vi "OnDataChange.vi"(0 "GRMActor in":refnum<class "FlatField.lvclass">, 1 "DataExchange":T1, 3 "error in (no error)":errorcluster) -> (7 "GRMActor out":refnum<class "FlatField.lvclass">, 10 "error out":errorcluster)   [LabVIEW 2020, in "FlatField.lvlib" / "FlatField.lvclass"]
uses:
  FlatField.lvclass
  Hardware Abstraction Layer/Component/Device/Device/DataExchange.ctl
  Displayer/Displayer/FlatField Method.ctl
  FlatField.lvclass/FlatField.ctl
  Interface/DataListener Messages/OnDataChange Msg/OnDataChange Msg.lvclass/OnDataChange Msg.ctl
  <vilib>/ActorFramework/Message Enqueuer/Message Enqueuer.lvclass/Message Enqueuer.ctl
  FlatField Status.ctl
  <vilib>/ActorFramework/Message Enqueuer/Enqueue.vi
  Interface/DataListener Messages/OnDataChange Msg/OnDataChange Msg.lvclass
  C:/Program Files/National Instruments/LabVIEW 2020/vi.lib/ActorFramework/Message/Message.lvclass
  <vilib>/ActorFramework/Message Priority Queue/Priority Enqueue.vi
  Hardware Abstraction Layer/Component/GenericActor/GenericActor/GenericActor.lvclass
  Interface/DataListener/DataListener.lvclass
  <vilib>/vision/NI_Vision_Development_Module.lvlib
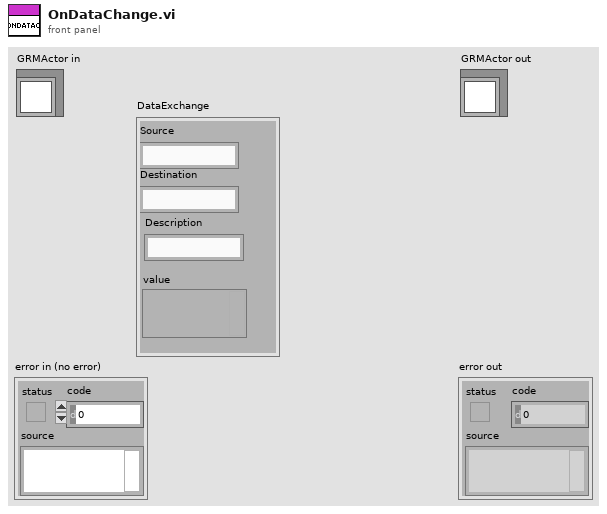
[diagram p1: front panel]
types:
  T1 = typedef "DataListener.lvclass/DataExchange.ctl" = cluster{"Source":string, "Destination":string, "Description":string, "value":variant}
  T2 = typedef "FlatField.lvlib/FlatField.lvclass/FlatField Method.ctl" = i32
  T3 = typedef "IMAQ Image.ctl" = refnum<image>
  T4 = typedef "FlatField.lvlib/FlatField.lvclass/FlatField Status.ctl" = i32
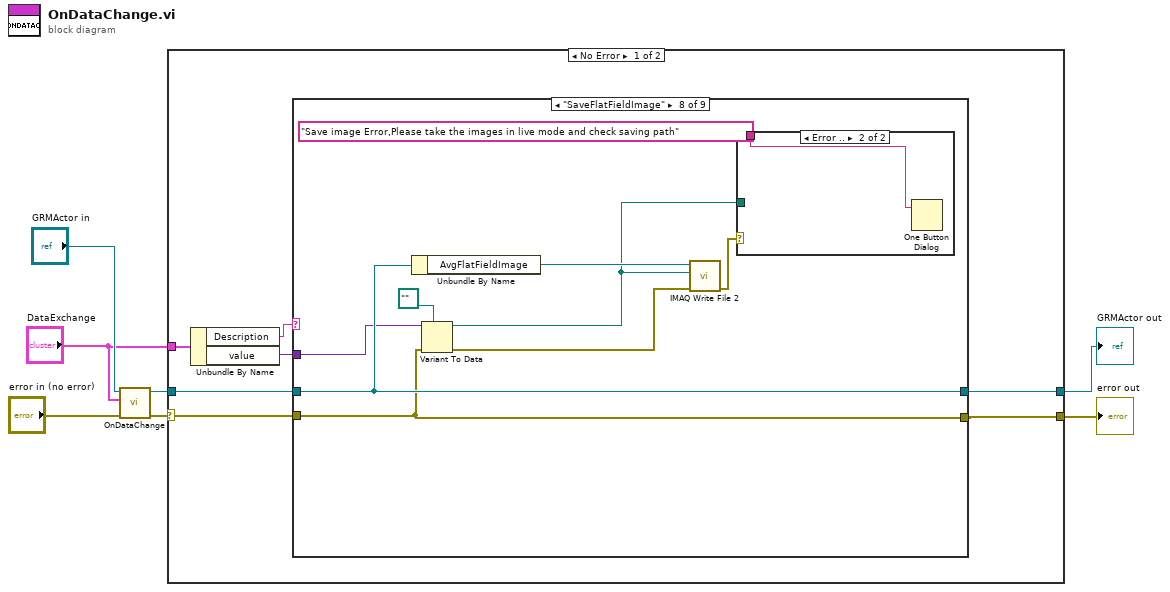
[diagram p0: block diagram]
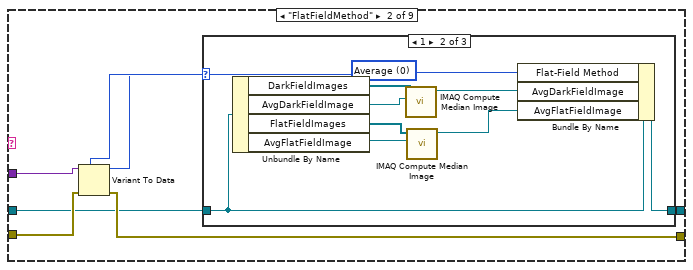
[diagram p3: hidden frame]
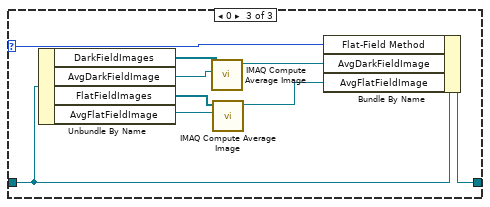
[diagram p5: hidden frame]
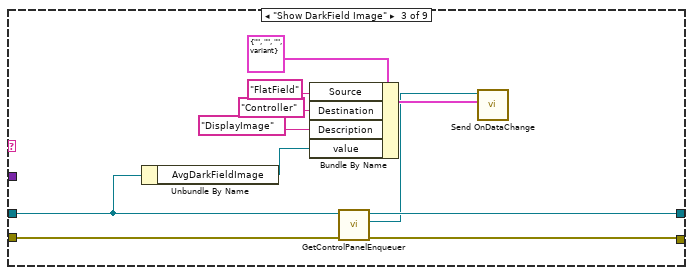
[diagram p6: hidden frame]
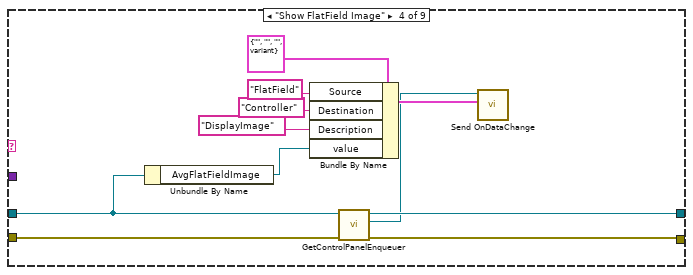
[diagram p7: hidden frame]
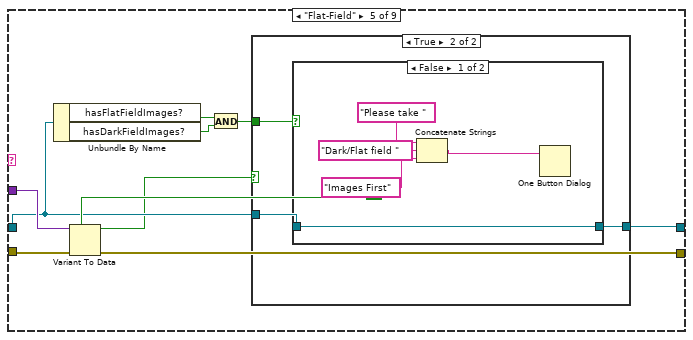
[diagram p8: hidden frame]
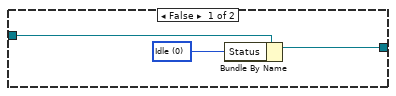
[diagram p9: hidden frame]
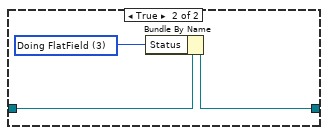
[diagram p10: hidden frame]
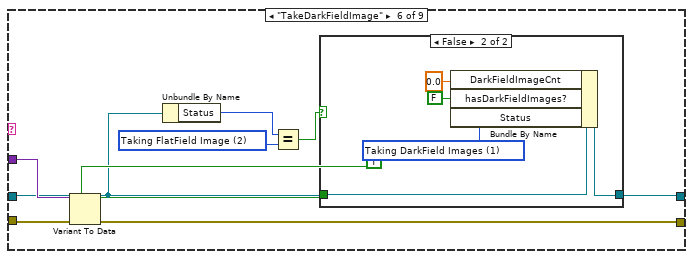
[diagram p11: hidden frame]
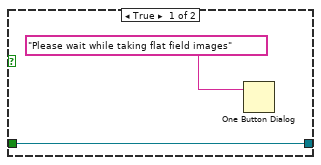
[diagram p12: hidden frame]
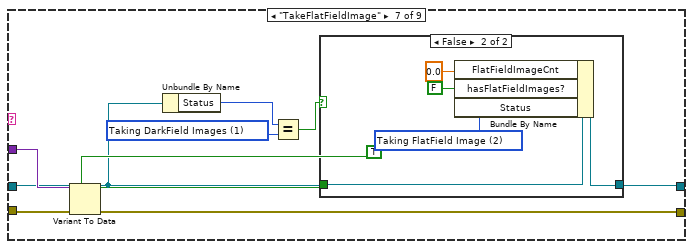
[diagram p13: hidden frame]
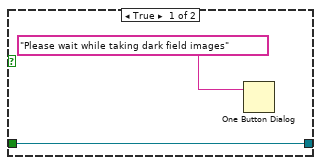
[diagram p14: hidden frame]
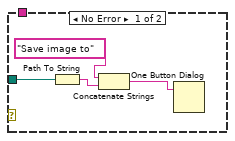
[diagram p15: hidden frame]
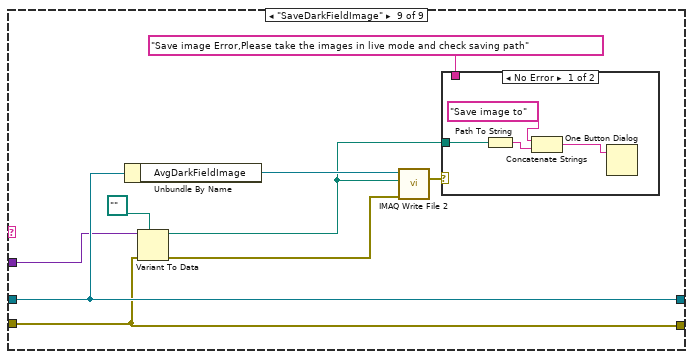
[diagram p16: hidden frame]
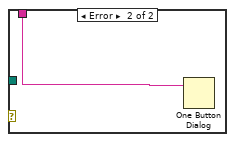
[diagram p17: hidden frame]
diagram:
  n1 = call-parent "OnDataChange.vi"("GRMActor in"="GRMActor in", "DataExchange"="DataExchange", "error in (no error)"="error in (no error)") -> ("GRMActor out"=w3:refnum<class "FlatField.lvclass">, "error out"=w5:errorcluster)  [unwired: 6 in]
  n2 = case shown="No Error" w5 {
    selector: w5 -> [w10 w151]
    tunnel: [w9 w151] -> w4
    tunnel: [w8 w152] -> w2
    tunnel: w3 -> [w11 w152]
    tunnel: "DataExchange" -> [w14 _]
    frame No Error {
      n3 = Unbundle By Name(w14) -> ("Description"=w13:string, "value"=w12:variant)
      n4 = case shown="\"SaveFlatFieldImage\"" w13 {
        tunnel: w12 -> [_ w20 _ _ w72 w96 w113 w129 w143]
        tunnel: [w16 w19 w46 w57 w70 w94 w111 w131 w145] -> w8
        tunnel: w11 -> [w16 w18 w44 w55 w69 w92 w109 w131 w145]
        tunnel: [w15 w22 w47 w58 w73 w97 w114 w125 w139] -> w9
        tunnel: w10 -> [w15 w23 w53 w64 w74 w98 w115 w125 w139]
        frame Default {
        }
        frame "FlatFieldMethod" {
          w21 = T2 0 items=["Average", "Median"] ("Flat-Field Method")
          n5 = Variant To Data(error in=w23, type=w21, Variant=w20) -> (data=w17:T2, error out=w22:errorcluster)
          n6 = case shown="1" w17 {
            selector: w17 -> [_ w31 w40]
            tunnel: [w24 w33 w42] -> w19
            tunnel: w18 -> [w24 w32 w41]
            frame Default {
            }
            frame 1 {
              n7 = Unbundle By Name(w32) -> ("DarkFieldImages"=w30:T3[], "AvgDarkFieldImage"=w29:T3, "FlatFieldImages"=w27:T3[], "AvgFlatFieldImage"=w26:T3)
              n8 = call "IMAQ Compute Median Image"("Image Dst"=w29, "Images"=w30) -> ("Image Dst Out"=w28:T3)  [unwired: 8 in, 1 out]
              n9 = call "IMAQ Compute Median Image"("Image Dst"=w26, "Images"=w27) -> ("Image Dst Out"=w25:T3)  [unwired: 8 in, 1 out]
              n10 = Bundle By Name(cluster=w32, "Flat-Field Method"=w31, "AvgDarkFieldImage"=w28, "AvgFlatFieldImage"=w25) -> (w33:refnum<class "FlatField.lvclass">)
            }
            frame 0 {
              n11 = Unbundle By Name(w41) -> ("DarkFieldImages"=w39:T3[], "AvgDarkFieldImage"=w38:T3, "FlatFieldImages"=w36:T3[], "AvgFlatFieldImage"=w35:T3)
              n12 = call "IMAQ Compute Average Image"("Image Dst"=w38, "Images"=w39) -> ("Image Dst Out"=w37:T3)  [unwired: 8 in, 1 out]
              n13 = call "IMAQ Compute Average Image"("Image Dst"=w35, "Images"=w36) -> ("Image Dst Out"=w34:T3)  [unwired: 8 in, 1 out]
              n14 = Bundle By Name(cluster=w41, "Flat-Field Method"=w40, "AvgDarkFieldImage"=w37, "AvgFlatFieldImage"=w34) -> (w42:refnum<class "FlatField.lvclass">)
            }
          }
        }
        frame "Show DarkField Image" {
          n15 = Unbundle By Name(w44) -> ("AvgDarkFieldImage"=w43:T3)
          n16 = Bundle By Name(cluster=T1 {"Source"="", "Destination"="", "Description"="", "value"=variant} ("DataExchange"), "Source"="FlatField", "Destination"="Controller", "Description"="DisplayImage", "value"=w43) -> (w51:T1)
          n17 = call-dynamic "GetControlPanelEnqueuer.vi"("error in (no error)"=w53, "GRMActor in"=w44) -> ("error out"=w47:errorcluster, "ControlViewEnqueuer"=w45:refnum<class "Message Enqueuer.lvclass">, "GRMActor out"=w46:refnum<class "FlatField.lvclass">)  [unwired: 7 in]
          n18 = call "Send OnDataChange.vi"("DataExchange"=w51, "Message Enqueuer"=w45) -> ()  [unwired: 8 in, 2 out]
        }
        frame "Show FlatField Image" {
          n19 = Unbundle By Name(w55) -> ("AvgFlatFieldImage"=w54:T3)
          n20 = Bundle By Name(cluster=T1 {"Source"="", "Destination"="", "Description"="", "value"=variant} ("DataExchange"), "Source"="FlatField", "Destination"="Controller", "Description"="DisplayImage", "value"=w54) -> (w62:T1)
          n21 = call-dynamic "GetControlPanelEnqueuer.vi"("error in (no error)"=w64, "GRMActor in"=w55) -> ("error out"=w58:errorcluster, "ControlViewEnqueuer"=w56:refnum<class "Message Enqueuer.lvclass">, "GRMActor out"=w57:refnum<class "FlatField.lvclass">)  [unwired: 7 in]
          n22 = call "Send OnDataChange.vi"("DataExchange"=w62, "Message Enqueuer"=w56) -> ()  [unwired: 8 in, 2 out]
        }
        frame "Flat-Field" {
          n23 = Unbundle By Name(w69) -> ("hasFlatFieldImages?"=w68:bool, "hasDarkFieldImages?"=w67:bool)
          n24 = Variant To Data(error in=w74, type=TRUE ("Boolean"), Variant=w72) -> (data=w65:bool, error out=w73:errorcluster)
          n25 = And(x=w68, y=w67) -> (x .and. y?=w66:bool)
          n26 = case shown="True" w65 {
            tunnel: [w76 w80] -> w70
            tunnel: w69 -> [w77 w79]
            tunnel: w66 -> [_ w78]
            frame False {
              w75 = T4 0 items=["Idle", "Taking DarkField Images", "Taking FlatField Image", "Doing FlatField", ""] ("Flat-Field Status")
              n27 = Bundle By Name(cluster=w77, "Status"=w75) -> (w76:refnum<class "FlatField.lvclass">)
            }
            frame True {
              n28 = case shown="False" w78 {
                tunnel: w79 -> [w81 w88]
                tunnel: [w81 w87] -> w80
                frame False {
                  n29 = Concatenate Strings("Please take " ("message"), "Dark/Flat field " ("string"), "Images First" ("string")) -> (w84:string)
                  n30 = One Button Dialog(message=w84) -> ()  [unwired: 1 in, 1 out]
                }
                frame True {
                  w86 = T4 3 items=["Idle", "Taking DarkField Images", "Taking FlatField Image", "Doing FlatField", ""] ("Flat-Field Status")
                  n31 = Bundle By Name(cluster=w88, "Status"=w86) -> (w87:refnum<class "FlatField.lvclass">)
                }
              }
            }
          }
        }
        frame "TakeDarkFieldImage" {
          w90 = T4 2 items=["Idle", "Taking DarkField Images", "Taking FlatField Image", "Doing FlatField", ""] ("y")
          n32 = Variant To Data(error in=w98, type=TRUE ("Boolean"), Variant=w96) -> (data=w93:bool, error out=w97:errorcluster)
          n33 = Unbundle By Name(w92) -> ("Status"=w91:T4)
          n34 = Equal?(x=w91, y=w90) -> (x = y?=w89:bool)
          n35 = case shown="False" w89 {
            tunnel: w92 -> [w100 w101]
            tunnel: [w100 w105] -> w94
            tunnel: w93 -> [_ _]
            frame True {
              n36 = One Button Dialog(message="Please wait while taking flat field images") -> ()  [unwired: 1 in, 1 out]
            }
            frame False {
              w102 = T4 1 items=["Idle", "Taking DarkField Images", "Taking FlatField Image", "Doing FlatField", ""] ("Flat-Field Status")
              n37 = Bundle By Name(cluster=w101, "DarkFieldImageCnt"=0.0, "hasDarkFieldImages?"=FALSE, "Status"=w102) -> (w105:refnum<class "FlatField.lvclass">)
            }
          }
        }
        frame "TakeFlatFieldImage" {
          w107 = T4 1 items=["Idle", "Taking DarkField Images", "Taking FlatField Image", "Doing FlatField", ""] ("y")
          n38 = Variant To Data(error in=w115, type=TRUE ("Boolean"), Variant=w113) -> (data=w110:bool, error out=w114:errorcluster)
          n39 = Unbundle By Name(w109) -> ("Status"=w108:T4)
          n40 = Equal?(x=w108, y=w107) -> (x = y?=w106:bool)
          n41 = case shown="False" w106 {
            tunnel: w109 -> [w117 w118]
            tunnel: [w117 w122] -> w111
            tunnel: w110 -> [_ _]
            frame True {
              n42 = One Button Dialog(message="Please wait while taking dark field images") -> ()  [unwired: 1 in, 1 out]
            }
            frame False {
              w119 = T4 2 items=["Idle", "Taking DarkField Images", "Taking FlatField Image", "Doing FlatField", ""] ("Flat-Field Status")
              n43 = Bundle By Name(cluster=w118, "FlatFieldImageCnt"=0.0 ("DarkFieldImageCnt"), "hasFlatFieldImages?"=FALSE ("hasDarkFieldImages?"), "Status"=w119) -> (w122:refnum<class "FlatField.lvclass">)
            }
          }
        }
        frame "SaveFlatFieldImage" {
          n44 = Unbundle By Name(w131) -> ("AvgFlatFieldImage"=w130:T3)
          n45 = Variant To Data(error in=w125, type=path "" ("Path"), Variant=w129) -> (data=w126:path, error out=w127:errorcluster)
          n46 = call-poly "IMAQ Write File 2"("error in (no error)"=w127, "File Path"=w126, "Image"=w130) -> ("error out"=w124:errorcluster)  [unwired: 7 in, 1 out]
          n47 = case shown="Error .." w124 {
            tunnel: w126 -> [w135 _]
            tunnel: "Save image Error,Please take the images in live mode and check saving path" ("message") -> [_ w136]
            frame No Error {
              n48 = Path To String(path=w135) -> (string=w133:string)
              n49 = Concatenate Strings("Save image to" ("message"), w133) -> (w132:string)
              n50 = One Button Dialog(message=w132) -> ()  [unwired: 1 in, 1 out]
            }
            frame Error {
              n51 = One Button Dialog(message=w136) -> ()  [unwired: 1 in, 1 out]
            }
          }
        }
        frame "SaveDarkFieldImage" {
          n52 = Unbundle By Name(w145) -> ("AvgDarkFieldImage"=w144:T3)
          n53 = Variant To Data(error in=w139, type=path "" ("Path"), Variant=w143) -> (data=w140:path, error out=w141:errorcluster)
          n54 = call-poly "IMAQ Write File 2"("error in (no error)"=w141, "File Path"=w140, "Image"=w144) -> ("error out"=w138:errorcluster)  [unwired: 7 in, 1 out]
          n55 = case shown="No Error" w138 {
            tunnel: w140 -> [w149 _]
            tunnel: "Save image Error,Please take the images in live mode and check saving path" ("message") -> [_ w150]
            frame No Error {
              n56 = Path To String(path=w149) -> (string=w147:string)
              n57 = Concatenate Strings("Save image to" ("message"), w147) -> (w146:string)
              n58 = One Button Dialog(message=w146) -> ()  [unwired: 1 in, 1 out]
            }
            frame Error {
              n59 = One Button Dialog(message=w150) -> ()  [unwired: 1 in, 1 out]
            }
          }
        }
      }
    }
    frame Error {
    }
  }
  "error out" <- w4
  "GRMActor out" <- w2
